vi "Set Inst Vel Param.vi"(8 "error in (no error)":errorcluster, 10 "Inst Vel":i32, 11 "FujiMotor in":refnum<class "FujiMotor.lvclass">) -> (0 "error out":errorcluster, 3 "FujiMotor out":refnum<class "FujiMotor.lvclass">)   [LabVIEW 2014, in "ALPHA5 RS485.lvlib" / "FujiMotor.lvclass"]
uses:
  FujiMotor.lvclass
  FujiMotor.lvclass/FujiMotor.ctl
  ALPHA5 RS485.lvlib
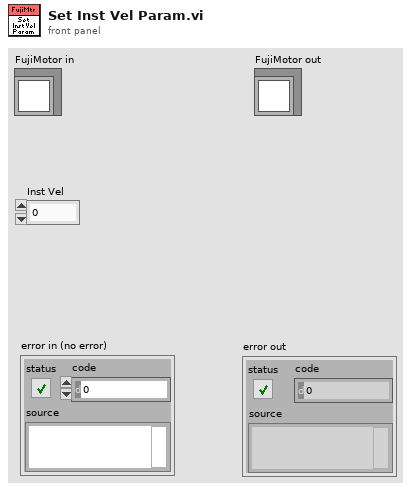
[diagram p1: front panel]
types:
  T1 = typedef "ALPHA5 RS485.lvlib/Port Selection Info.ctl" = cluster{"Port Name":refnum<visa-resource-name>, "Amplifier Num":u8, "Baud Rate":u32, "Char Formation":enum16{"0", "1", "2", "3", "4", "5"}}
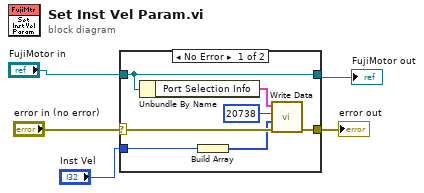
[diagram p0: block diagram]
diagram:
  n1 = case shown="No Error" "error in (no error)" {
    selector: "error in (no error)" -> [w11 w13]
    tunnel: "FujiMotor in" -> [w6 w14]
    tunnel: "Inst Vel" -> [w9 _]
    tunnel: [w7 w13] -> w3
    tunnel: [w6 w14] -> w2
    frame No Error {
      n2 = Unbundle By Name(w6) -> ("Port Selection Info"=w12:T1)
      n3 = Build Array(w9) -> (w8:i32[])
      n4 = call "Write Data.vi"("error in (no error)"=w11, "Data"=w8, "Address"=u16 20738, "Port Selection Info In"=w12) -> ("error out"=w7:errorcluster)  [unwired: 6 in, 1 out]
    }
    frame Error {
    }
  }
  "FujiMotor out" <- w2
  "error out" <- w3
